vi "Not A Listener.vi"(1 "listener":T1) -> (0 "Not a Listener?":bool)   [LabVIEW 2013, in "libssh2.lvlib"]
doc: "Returns TRUE if <B>listener</B> is not a listener. Otherwise, FALSE."
uses:
  libssh2.lvlib
  Listener Refnum.ctl
  Listener Refnum Data.ctl
  Session Refnum.ctl
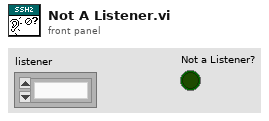
[diagram p1: front panel]
types:
  T1 = typedef "libssh2.lvlib/Listener Refnum.ctl" = refnum<k1>
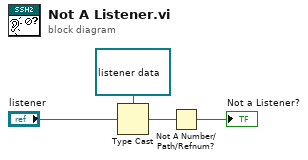
[diagram p0: block diagram]
diagram:
  n1 = Type Cast(type=refnum<data-value> refnum ("data value reference"), x="listener") -> (*(type *) &x=w3:refnum<data-value>)
  n2 = Not A Number/Path/Refnum?(number/path/refnum=w3) -> (NaN/Path/Refnum?=→"Not a Listener?":bool)
